vi "Starting_point.vi"() -> ()   [LabVIEW 2021]
uses:
  <instrlib>/E5270_Paramater_analyser/E5270_Paramater_analyser.lvlib
panel:
  out "SMU3 Terminal":string
  out "SMU2 Terminal":string
  in  "SMU1 Terminal":string(combo)
  in  "Estimated Sample Dimensions":string
  in  "Sample Information":string
  in  "User":string
  in  "error in (no error)":errorcluster
  out "VISA resource name out":refnum<visa-resource-name>
  out "error out":errorcluster
  in  "VISA resource name":refnum<visa-resource-name>="PA"
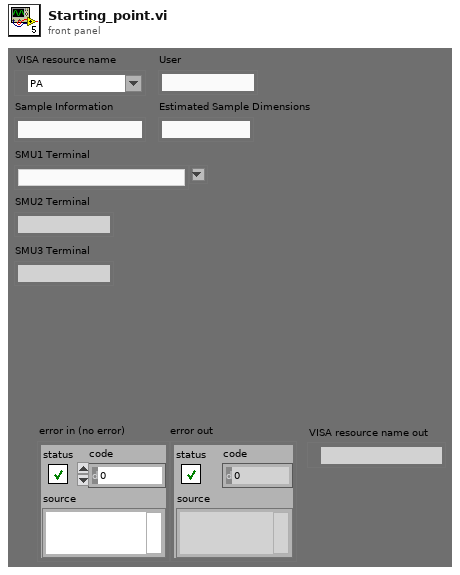
[diagram p1: front panel]
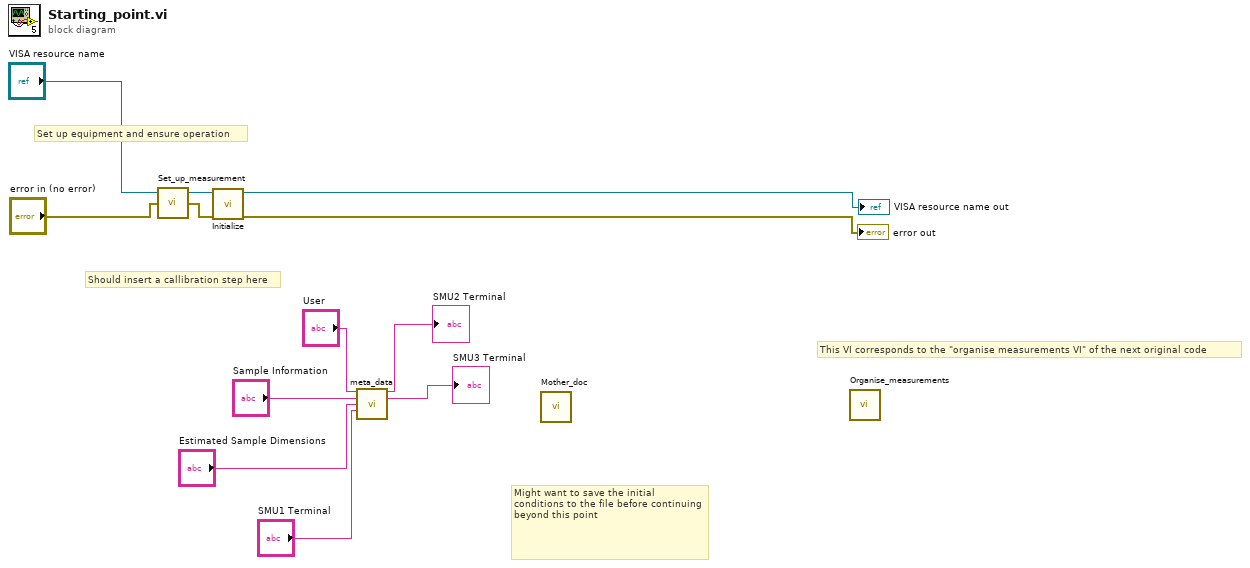
[diagram p0: block diagram]
diagram:
  # "This VI corresponds to the \"organise measurements VI\" of the next original code"
  # "Might want to save the initial conditions to the file before continuing beyond this point"
  # "Should insert a callibration step here"
  # "Set up equipment and ensure operation"
  n1 = call "Set_up_measurement.vi"("error in (no error)"="error in (no error)", "VISA resource name"="VISA resource name") -> ("error out"=w10:errorcluster, "VISA resource name out"=w9:refnum<visa-resource-name>)  [unwired: 2 in]
  n2 = call <instrlib>:"Initialize.vi"("error in (no error)"=w10, "VISA resource name"=w9) -> ("error out"=→"error out":errorcluster, "VISA resource name out"=→"VISA resource name out":refnum<visa-resource-name>)  [unwired: 7 in, 1 out]
  n3 = call "meta_data.vi"("User"="User", "Sample Information"="Sample Information", "Estimated Sample Dimensions"="Estimated Sample Dimensions", "SMU1 Terminal"="SMU1 Terminal") -> ("SMU2 Terminal"=→"SMU2 Terminal":string, "SMU3 Terminal"=→"SMU3 Terminal":string)  [unwired: 10 in]
  n4 = call "Mother_doc.vi"() -> ()  [unwired: 28 in]
  n5 = call "Organise_measurements.vi"() -> ()  [unwired: 20 in]
